vi "Phase word to Frequency.vi"(6 "Time delay":dbl=-2.0, 7 "Phase word":u64=1717987 format="0x%x (%d) 0b%b", 9 "DDS modulus":i64=4294967296 format="0x%x (%d)", 10 "DDS clock":dbl=125000000.0 format="%_13p", 11 "Frequency word":u64=1717987 format="0x%x (%d) 0b%b") -> (1 "Points per sine wave":u64, 2 "Actual frequency":dbl format="%#_12pHz", 4 "Syncronous":bool, 5 "Phase":dbl format="%#_gdeg")   [LabVIEW 2019]
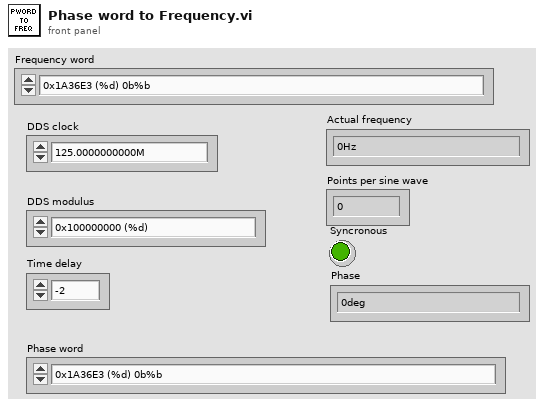
[diagram p1: front panel]
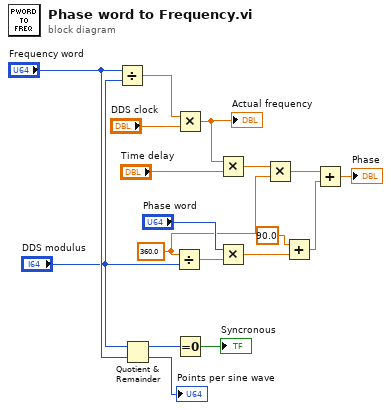
[diagram p0: block diagram]
diagram:
  w3 = 360.0
  n1 = Divide(x="Frequency word", y="DDS modulus") -> (x/y=w18:dbl)
  n2 = Quotient & Remainder(x="DDS modulus", y="Frequency word") -> (x-y*floor(x/y)=w17:u64, floor(x/y)=→"Points per sine wave":u64)
  n3 = Divide(x=w3, y="DDS modulus") -> (x/y=w14:dbl)
  n4 = Multiply(x=w18, y="DDS clock") -> (x*y=w5:dbl)
  "Actual frequency" <- w5
  n5 = Equal To 0?(x=w17) -> (x = 0?=→"Syncronous":bool)
  n6 = Multiply(x=w5, y="Time delay") -> (x*y=w4:dbl)
  n7 = Multiply(x="Phase word", y=w14) -> (x*y=w11:dbl)
  n8 = Multiply(x=w4, y=w3) -> (x*y=w1:dbl)
  n9 = Add(x=90.0, y=w11) -> (x+y=w10:dbl)
  n10 = Add(x=w1, y=w10) -> (x+y=→"Phase":dbl)
